vi "generate default line.vi"(8 "error in":errorcluster, 10 "last line":T1, 11 "operations table":T2) -> (0 "error out":errorcluster, 2 "line":T1)   [LabVIEW 2013, in "Modbus Module editor node.lvclass"]
doc: "Platypus Framework 1.0.1.65\nNI Systems Engineering - National Instruments"
uses:
  Modbus Module editor node.lvclass
  table reference.ctl
  table line.ctl
  module/module channel/Modbus Module Channel.lvclass
  <vilib>/NI/Tag Bus/tag/tag descriptor.lvclass/tag descriptor.ctl
  module/module channel/Modbus Module Channel.lvclass/Modbus Module Channel.ctl
  <vilib>/NI/Tag Bus/tag/Data Type.ctl
  module/module channel/data bank type.ctl
  <vilib>/NI/Tag Bus/tag/read tag name.vi
  <vilib>/NI/Tag Bus/tag/read data type.vi
  module/module channel/Read modbus type.vi
  <vilib>/NI/Tag Bus/tag/write data type.vi
  module/module channel/Write modbus type.vi
  module/module channel/Write starting address.vi
  <vilib>/NI/Tag Bus/tag/write tag name.vi
  <vilib>/NI/Tag Bus/tag/tag descriptor.lvclass
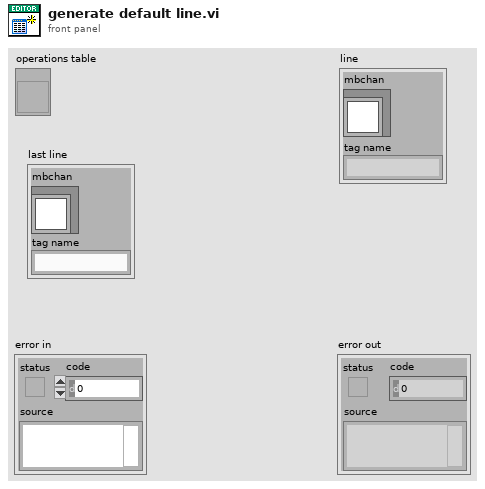
[diagram p1: front panel]
types:
  T1 = typedef "Modbus Module editor node.lvclass/table line.ctl" = cluster{"mbchan":refnum<class "Modbus Module Channel.lvclass">, "tag name":string}
  T2 = typedef "Modbus Module editor node.lvclass/table reference.ctl" = refnum<vi>
  T3 = typedef "tag bus.lvlib/tag descriptor.lvclass/Data Type.ctl" = enum16{"Double", "Single", "I64", "I32", "I16", "I8", "U64", "U32", "U16", "U8", "Boolean", "String", "Array of Double", "Array of Single", "Array of I64", "Array of I32", "Array of I16", "Array of I8", "Array of U64", "Array of U32", "Array of U16", "Array of U8", "Array of Boolean", "Array of String"}
  T4 = typedef "Modbus Module Channel.lvclass/data bank type.ctl" = enum16{"coils", "discrete inputs", "input registers", "holding registers"}
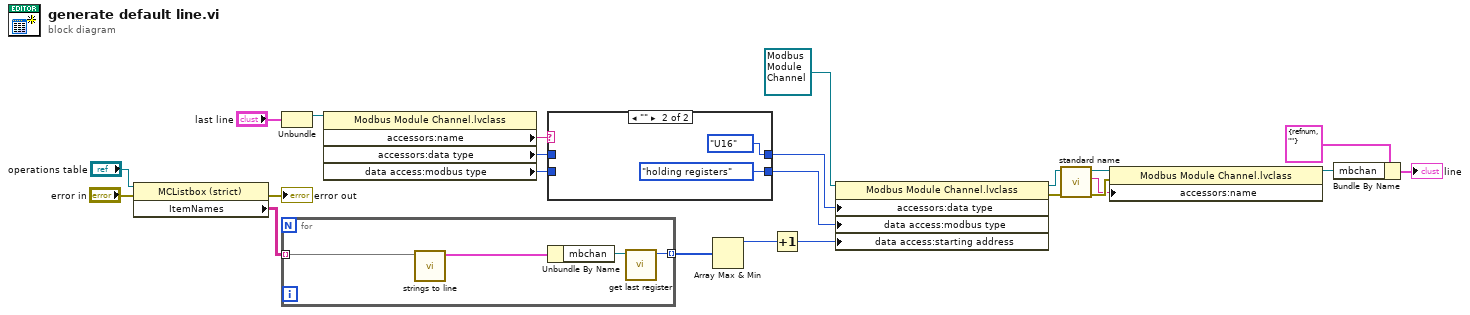
[diagram p0: block diagram]
diagram:
  n1 = property class="MCListbox (strict)"(reference="operations table", error in="error in") -> (error out=→"error out":errorcluster, "ItemNames"=w20:string[][])  [unwired: 1 out]
  n2 = Unbundle("last line") -> ("mbchan"=w15:refnum<class "Modbus Module Channel.lvclass">)  [unwired: 1 out]
  n3 = for {
    tunnel: w20 -> [w27] mode=indexing
    tunnel: [w24] -> w9 mode=indexing
    n4 = call "strings to line.vi"("strings"=w27) -> ("line"=w26:T1)  [unwired: 10 in]
    n5 = Unbundle By Name(w26) -> ("mbchan"=w25:refnum<class "Modbus Module Channel.lvclass">)
    n6 = call "get last register.vi"("Modbus Module Channel in"=w25) -> ("last element"=w24:i32)  [unwired: 10 in]
  }
  n7 = property class="Modbus Module Channel.lvclass"(reference=w15) -> ("accessors:name"=w14:string, "accessors:data type"=w11:T3, "data access:modbus type"=w10:T4)  [unwired: 1 in, 2 out]
  n8 = case shown="\"\"" w14 {
    tunnel: [w29 Data_Type."U16" ("data type")] -> w13
    tunnel: [w28 data_bank_type."holding registers" ("modbus type")] -> w12
    tunnel: w11 -> [w29 _]
    tunnel: w10 -> [w28 _]
    frame Default {
    }
    frame "" {
    }
  }
  n9 = Array Max & Min(array=w9) -> (max value=w8:i32)  [unwired: 3 out]
  n10 = Increment(x=w8) -> (x+1=w7:i32)
  n11 = property class="Modbus Module Channel.lvclass"(reference=refnum<class "Modbus Module Channel.lvclass"> refnum ("Modbus Module Channel"), "accessors:data type"=w13, "data access:modbus type"=w12, "data access:starting address"=w7) -> (reference out=w4:refnum<class "Modbus Module Channel.lvclass">, error out=w3:errorcluster)  [unwired: 1 in]
  n12 = call "standard name.vi"("error in"=w3, "Modbus Module Channel in"=w4) -> ("error out"=w2:errorcluster, "standard name"=w1:string, "Modbus Module Channel out"=w5:refnum<class "Modbus Module Channel.lvclass">)  [unwired: 7 in]
  n13 = property class="Modbus Module Channel.lvclass"(reference=w5, error in=w2, "accessors:name"=w1) -> (reference out=w6:refnum<class "Modbus Module Channel.lvclass">)  [unwired: 1 out]
  n14 = Bundle By Name(cluster=T1 {"mbchan"=refnum, "tag name"=""} ("line"), "mbchan"=w6) -> (→"line":T1)
